vi "获取量程参数存入关键参数.vi"(7 "关键参数变更":bool, 8 "error in (no error)":errorcluster caption="错误输入（无错误）", 9 "量程":u16, 10 "flowid":u16, 11 "id":u16) -> (0 "error out":errorcluster caption="错误输出")   [LabVIEW 2016, in "斯坦道总磷.lvlib"]
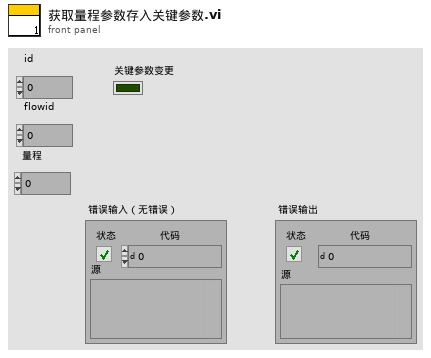
[diagram p1: front panel]
types:
  T1 = cluster{"运行模式":enum16{"维护模式", "常规模式", "应急模式", "质控模式", "性能测试"}, "质控频次":enum16{"关闭", "每天", "星期一", "星期二", "星期三", "星期四", "星期五", "星期六", "星期日"}, "空白核查时间":u16, "跨度核查时间":u16, "测量间隔":u16}
  T2 = cluster{"总磷":dbl, "总氮":dbl, "氨氮":dbl, "磷酸盐":dbl, "硝氮":dbl, "亚硝氮":dbl, "硅酸盐":dbl, "硫化物":dbl, "COD":dbl, "氟化物":dbl, "CODMn":dbl}
  T3 = cluster{"标液浓度1":dbl, "测量吸光度1":dbl, "样品1启用":bool, "标液浓度2":dbl, "测量吸光度2":dbl, "样品2启用":bool, "标液浓度3":dbl, "测量吸光度3":dbl, "样品3启用":bool, "标液浓度4":dbl, "测量吸光度4":dbl, "样品4启用":bool, "标液浓度5":dbl, "测量吸光度5":dbl, "样品5启用":bool, "模型":enum32{"线性", "多项式"}, "精度":dbl, "XY图":cluster{"X Values":dbl[], "Y Values":dbl[]}[], "拟合公式":string, "r^2":dbl, "标样一校准时间":timestamp, "标样二校准时间":timestamp, "标样三校准时间":timestamp, "标样四校准时间":timestamp, "标样五校准时间":timestamp, "二次方程":cluster{"c":dbl, "x":dbl, "x^2":dbl}, "标定时间":timestamp}
  T4 = cluster{"测量精度":u16, "检出限":dbl, "上限":dbl, "下限":dbl, "阈值（低->高）":dbl, "阈值（高->低）":dbl, "稀释度":dbl}
  T5 = typedef "SingleStepTestV3.lvlib/SingleStepTestV3.lvclass/仪器版本.ctl" = enum16{"A版", "B版", "A1版"}
  T6 = typedef "斯坦道总磷.lvlib/V3 A版外设参数.ctl" = cluster{"泵类型":u8, "进样速度":u32, "出样速度":u32, "泵阀量":u8, "阀方向":u8, "光谱仪类型":u8, "光谱采样次数":u8, "氙灯次数":u8, "B":u16, "C":u16, "D":u16, "E":u16, "B_COD":u16, "C_COD":u16, "D_COD":u16, "E_COD":u16, "G":u16, "M":u16, "N":u16, "氨氮注射泵控温下限":sgl, "氨氮注射泵控温上限":sgl, "总氮注射泵控温下限":sgl, "总氮注射泵控温上限":sgl, "消解温度下限":sgl, "消解温度上限":sgl, "加热10s限值":sgl, "KP":sgl, "KI":sgl, "KD":sgl, "高温高压阀开阀温度":sgl, "总氮x公式0":u8, "总氮x公式1":sgl, "总氮x公式2":sgl, "总磷浊度稀释系数":sgl, "总磷浊度补偿权重1":sgl, "总磷浊度补偿权重2":sgl, "盐度系数":sgl, "氨氮补偿系数1":sgl, "氨氮补偿系数2":sgl}
  T7 = typedef "斯坦道总磷.lvlib/V3 B版外设参数.ctl" = cluster{"泵类型":u8, "注射泵正常速度":u32, "注射泵慢速":u32, "阀型号":u8, "res":u8, "光谱仪类型":u8, "光谱采样次数":u8, "氙灯次数":u8, "B":u16, "C":u16, "D":u16, "E":u16, "B_COD":u16, "C_COD":u16, "D_COD":u16, "E_COD":u16, "G":u16, "M":u16, "N":u16, "降温下限":sgl, "降温上限":sgl, "恒温温度下限":sgl, "恒温温度上限":sgl, "消解温度下限":sgl, "消解温度上限":sgl, "加热10s限值":sgl, "KP":sgl, "KI":sgl, "KD":sgl, "高温高压阀开阀温度":sgl, "总氮x公式0":u8, "总氮x公式1":sgl, "总氮x公式2":sgl, "总磷浊度稀释系数":sgl, "总磷浊度补偿权重1":sgl, "总磷浊度补偿权重2":sgl, "盐度系数":sgl, "氨氮补偿系数1":sgl, "氨氮补偿系数2":sgl, "缺试剂传感器阈值":u16}
  T8 = typedef "斯坦道总磷.lvlib/V3 A1版外设参数.ctl" = cluster{"泵类型":u8, "进样速度":u32, "出样速度":u32, "泵阀量":u8, "光谱仪类型":u8, "光谱采样次数":u8, "氙灯次数":u8, "B":u16, "C":u16, "D":u16, "E":u16, "B_COD":u16, "C_COD":u16, "D_COD":u16, "E_COD":u16, "G":u16, "M":u16, "N":u16, "氨氮注射泵控温下限":sgl, "氨氮注射泵控温上限":sgl, "总氮注射泵控温下限":sgl, "总氮注射泵控温上限":sgl, "消解温度下限":sgl, "消解温度上限":sgl, "加热10s限值":sgl, "高温高压阀开阀温度":sgl, "总氮x公式0":u8, "总氮x公式1":sgl, "总氮x公式2":sgl, "总磷浊度稀释系数":sgl, "总磷浊度补偿权重1":sgl, "总磷浊度补偿权重2":sgl, "盐度系数":sgl, "氨氮补偿系数1":sgl, "氨氮补偿系数2":sgl}
  T9 = cluster{"标液浓度1":dbl, "测量吸光度1":dbl, "样品1启用":bool, "标液浓度2":dbl, "测量吸光度2":dbl, "样品2启用":bool, "标液浓度3":dbl, "测量吸光度3":dbl, "样品3启用":bool, "标液浓度4":dbl, "测量吸光度4":dbl, "样品4启用":bool, "标液浓度5":dbl, "测量吸光度5":dbl, "样品5启用":bool, "模型":enum32{"线性", "多项式"}, "精度":dbl, "XY图":cluster{"X Values":dbl[], "Y Values":dbl[]}[], "拟合公式":string, "r^2":dbl, "标样一校准时间":timestamp, "标样二校准时间":timestamp, "标样三校准时间":timestamp, "标样四校准时间":timestamp, "标样五校准时间":timestamp, "二次方程":cluster{"c":dbl, "x":dbl, "x^2":dbl}, "标定时间":timestamp}[]
  T10 = typedef "斯坦道总磷.lvlib/关键参数.ctl" = cluster{"测量量程":sgl, "测量检出限":sgl, "测量精度":sgl, "测量间隔":sgl, "消解温度":sgl, "消解时长":sgl, "三项式系数":sgl, "二次多项式系数":sgl, "曲线斜率":sgl, "曲线截距":sgl, "线性相关系数":sgl, "空白校准时间":timestamp, "标样校准时间":timestamp, "测量信号值":sgl, "稀释倍数":sgl, "空白标定系数":sgl, "量程系数":sgl}
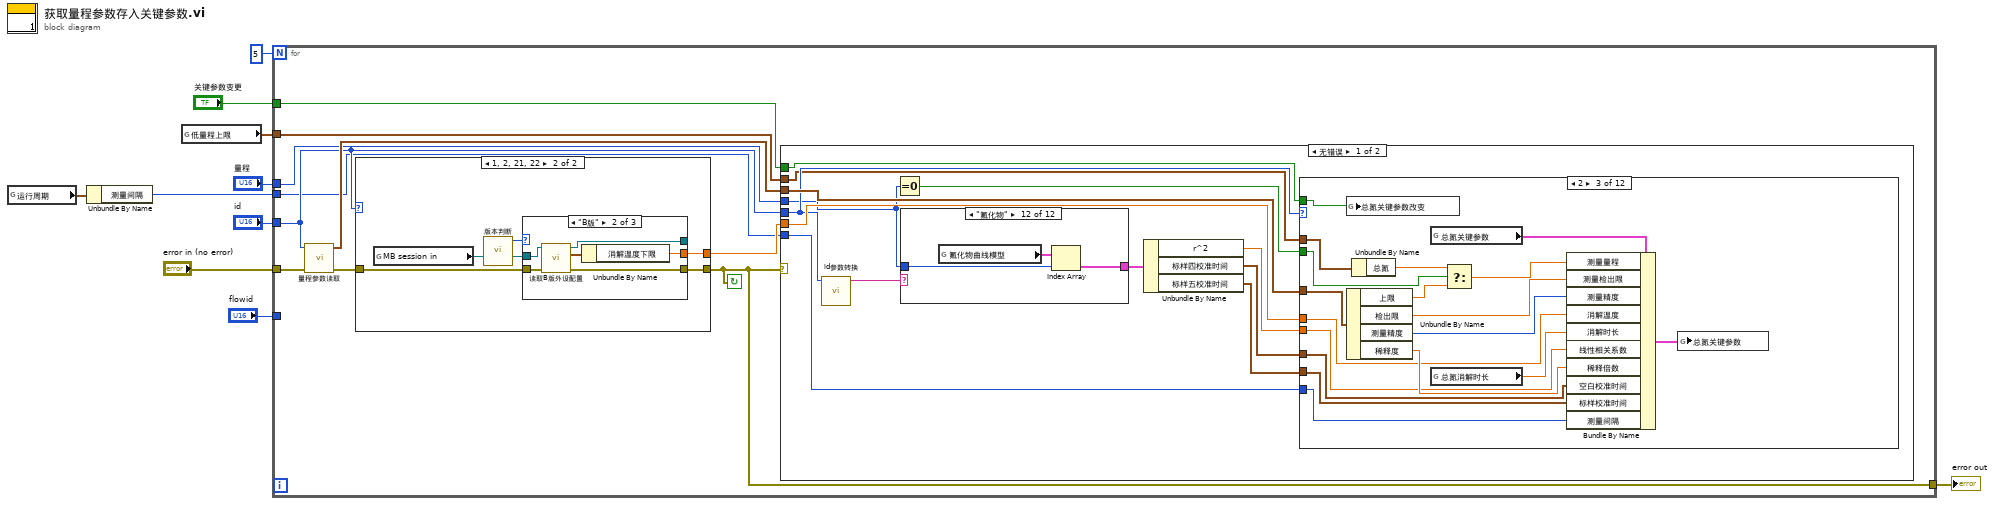
[diagram p0: block diagram]
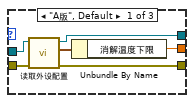
[diagram p3: hidden frame]
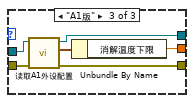
[diagram p4: hidden frame]
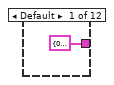
[diagram p5: hidden frame]
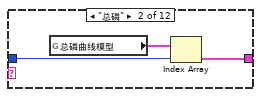
[diagram p6: hidden frame]
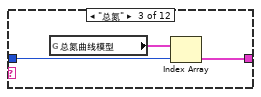
[diagram p7: hidden frame]
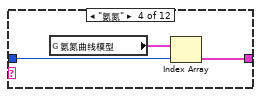
[diagram p8: hidden frame]
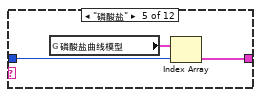
[diagram p9: hidden frame]
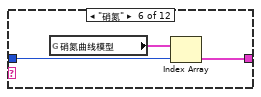
[diagram p10: hidden frame]
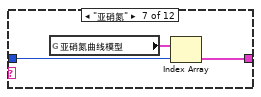
[diagram p11: hidden frame]
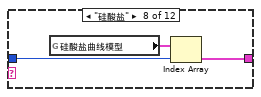
[diagram p12: hidden frame]
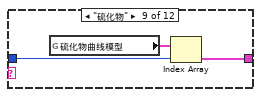
[diagram p13: hidden frame]
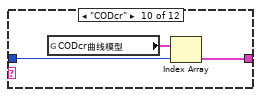
[diagram p14: hidden frame]
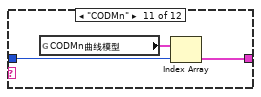
[diagram p15: hidden frame]
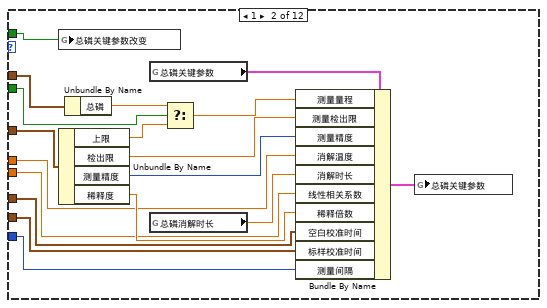
[diagram p17: hidden frame]
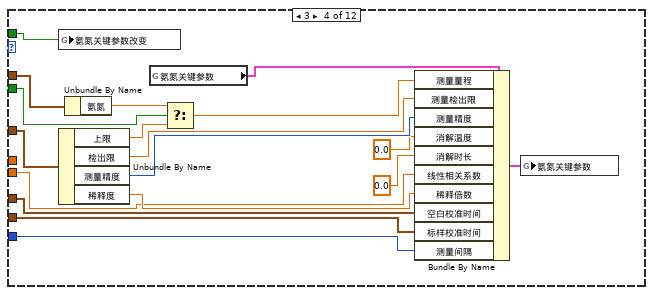
[diagram p18: hidden frame]
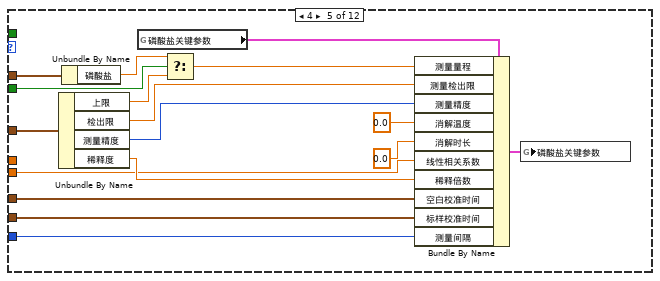
[diagram p19: hidden frame]
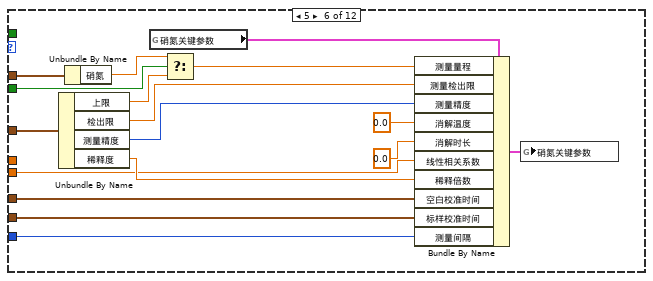
[diagram p20: hidden frame]
diagram:
  n1 = global read "总磷总氮断电保存全局变量.vi" "运行周期"() -> (w4:T1)
  n2 = Unbundle By Name(w4) -> ("测量间隔"=w3:u16)
  n3 = global read "总磷总氮断电保存全局变量.vi" "低量程上限"() -> (w2:T2)
  n4 = for {
    N: 5 -> [_]
    tunnel: "量程" -> [w18]
    tunnel: "flowid" -> [_]
    tunnel: "id" -> [w14]
    tunnel: "error in (no error)" -> [w15]
    tunnel: [w16] -> w5
    tunnel: w3 -> [w13]
    tunnel: w2 -> [w12]
    tunnel: "关键参数变更" -> [w11]
    stop <- w16 continue-if-true
    n5 = call "量程参数读取.vi"("error in (no error)"=w15, "测量参数"=w14) -> ("error out"=w17:errorcluster, "量程参数读取"=w20:T4)  [unwired: 8 in]
    n6 = case shown="1, 2, 21, 22" w14 {
      tunnel: [_ w24] -> w19
      tunnel: w17 -> [w21 w25]
      tunnel: [w21 w23] -> w16
      frame 0, Default {
      }
      frame 1, 2, 21, 22 {
        n7 = global read "VAR总磷总氮全局变量.vi" "MB session in"() -> (w26:refnum<class "MB_Master.lvclass">)
        n8 = call "版本判断.vi"() -> ("仪器版本"=w22:T5)  [unwired: 11 in]
        n9 = case shown="\"B版\"" w22 {
          tunnel: [w32 w38 w44] -> w23
          tunnel: [w30 w36 w42] -> w24
          tunnel: [w29 w35 w41] -> _
          tunnel: w26 -> [w28 w34 w40]
          tunnel: w25 -> [w27 w33 w39]
          frame "A版", Default {
            n10 = call "读取外设配置.vi"("error in (no error)"=w27, "MB session in"=w28) -> ("error out"=w32:errorcluster, "外设配置"=w31:T6, "MB session out"=w29:refnum<class "MB_Master.lvclass">)  [unwired: 7 in]
            n11 = Unbundle By Name(w31) -> ("消解温度下限"=w30:sgl)
          }
          frame "B版" {
            n12 = call "读取B版外设配置.vi"("error in (no error)"=w33, "MB session in"=w34) -> ("error out"=w38:errorcluster, "外设配置"=w37:T7, "MB session out"=w35:refnum<class "MB_Master.lvclass">)  [unwired: 7 in]
            n13 = Unbundle By Name(w37) -> ("消解温度下限"=w36:sgl)
          }
          frame "A1版" {
            n14 = call "读取A1外设配置.vi"("error in (no error)"=w39, "MB session in"=w40) -> ("error out"=w44:errorcluster, "外设配置"=w43:T8, "MB session out"=w41:refnum<class "MB_Master.lvclass">)  [unwired: 7 in]
            n15 = Unbundle By Name(w43) -> ("消解温度下限"=w42:sgl)
          }
        }
      }
    }
    n16 = case shown="无错误" w16 {
      tunnel: w20 -> [w57 _]
      tunnel: w19 -> [w56 _]
      tunnel: w14 -> [w50 _]
      tunnel: w18 -> [w47 _]
      tunnel: w13 -> [w49 _]
      tunnel: w12 -> [w48 _]
      tunnel: w11 -> [w45 _]
      frame No Error {
        n17 = call "id参数转换.vi"("id"=w50) -> ("table输出"=w55:string)  [unwired: 9 in, 1 out]
        n18 = Equal To 0?(x=w47) -> (x = 0?=w46:bool)
        n19 = case shown="\"氟化物\"" w55 {
          tunnel: w47 -> [_ w59 w62 w65 w68 w71 w74 w77 w80 w83 w86 w89]
          tunnel: [T3 {"标液浓度1"=0.0, "测量吸光度1"=0.0, "样品1启用"=FALSE, "标液浓度2"=0.0, "测量吸光度2"=0.0, "样品2启用"=FALSE, "标液浓度3"=0.0, "测量吸光度3"=0.0, "样品3启用"=FALSE, "标液浓度4"=0.0, "测量吸光度4"=0.0, "样品4启用"=FALSE, "标液浓度5"=0.0, "测量吸光度5"=0.0, "样品5启用"=FALSE, "模型"=enum."线性", "精度"=0.0, "XY图"=[], "拟合公式"="", "r^2"=0.0, "标样一校准时间"=timestamp(0 s since 1904-01-01), "标样二校准时间"=timestamp(0 s since 1904-01-01), "标样三校准时间"=timestamp(0 s since 1904-01-01), "标样四校准时间"=timestamp(0 s since 1904-01-01), "标样五校准时间"=timestamp(0 s since 1904-01-01), "二次方程"={"c"=0.0, "x"=0.0, "x^2"=0.0}, "标定时间"=timestamp(0 s since 1904-01-01)} ("总磷曲线模型") w60 w63 w66 w69 w72 w75 w78 w81 w84 w87 w90] -> w54
          frame Default {
          }
          frame "总磷" {
            n20 = global read "校准数据全局变量.vi" "总磷曲线模型"() -> (w61:T9)
            n21 = Index Array(array=w61, index=w59) -> (element=w60:T3)
          }
          frame "总氮" {
            n22 = global read "校准数据全局变量.vi" "总氮曲线模型"() -> (w64:T9)
            n23 = Index Array(array=w64, index=w62) -> (element=w63:T3)
          }
          frame "氨氮" {
            n24 = global read "校准数据全局变量.vi" "氨氮曲线模型"() -> (w67:T9)
            n25 = Index Array(array=w67, index=w65) -> (element=w66:T3)
          }
          frame "磷酸盐" {
            n26 = global read "校准数据全局变量.vi" "磷酸盐曲线模型"() -> (w70:T9)
            n27 = Index Array(array=w70, index=w68) -> (element=w69:T3)
          }
          frame "硝氮" {
            n28 = global read "校准数据全局变量.vi" "硝氮曲线模型"() -> (w73:T9)
            n29 = Index Array(array=w73, index=w71) -> (element=w72:T3)
          }
          frame "亚硝氮" {
            n30 = global read "校准数据全局变量.vi" "亚硝氮曲线模型"() -> (w76:T9)
            n31 = Index Array(array=w76, index=w74) -> (element=w75:T3)
          }
          frame "硅酸盐" {
            n32 = global read "校准数据全局变量.vi" "硅酸盐曲线模型"() -> (w79:T9)
            n33 = Index Array(array=w79, index=w77) -> (element=w78:T3)
          }
          frame "硫化物" {
            n34 = global read "校准数据全局变量.vi" "硫化物曲线模型"() -> (w82:T9)
            n35 = Index Array(array=w82, index=w80) -> (element=w81:T3)
          }
          frame "CODcr" {
            n36 = global read "校准数据全局变量.vi" "CODcr曲线模型"() -> (w85:T9)
            n37 = Index Array(array=w85, index=w83) -> (element=w84:T3)
          }
          frame "CODMn" {
            n38 = global read "校准数据全局变量.vi" "CODMn曲线模型"() -> (w88:T9)
            n39 = Index Array(array=w88, index=w86) -> (element=w87:T3)
          }
          frame "氟化物" {
            n40 = global read "校准数据全局变量.vi" "氟化物曲线模型"() -> (w91:T9)
            n41 = Index Array(array=w91, index=w89) -> (element=w90:T3)
          }
        }
        n42 = Unbundle By Name(w54) -> ("r^2"=w53:dbl, "标样四校准时间"=w52:timestamp, "标样五校准时间"=w51:timestamp)
        n43 = case shown="2" w50 {
          tunnel: w57 -> [_ w107 w125 w143 w160 w177 w194 w211 w228 w246 w264 w281]
          tunnel: w56 -> [_ w92 w110 _ _ _ _ _ _ w231 w249 w267]
          tunnel: w53 -> [_ w100 w120 w137 w152 w171 w188 w205 w220 w241 w259 w276]
          tunnel: w52 -> [_ w101 w119 w136 w154 w170 w187 w204 w222 w240 w258 w275]
          tunnel: w51 -> [_ w102 w118 w135 w153 w169 w186 w203 w221 w239 w257 w274]
          tunnel: w49 -> [_ w99 w117 w134 w151 w168 w185 w202 w219 w238 w256 w273]
          tunnel: w48 -> [_ w98 w115 w132 w149 w166 w183 w199 w217 w236 w254 w271]
          tunnel: w46 -> [_ w96 w114 w131 w148 w165 w182 w200 w216 w235 w253 w270]
          tunnel: w45 -> [_ w93 w111 w128 _ _ _ _ _ w232 w250 _]
          frame 0, Default {
          }
          frame 1 {
            n44 = global write "VAR总磷总氮全局变量.vi" "总磷关键参数改变"(w93) -> ()
            n45 = Unbundle By Name(w107) -> ("上限"=w95:dbl, "检出限"=w106:dbl, "测量精度"=w105:u16, "稀释度"=w103:dbl)
            n46 = Unbundle By Name(w98) -> ("总磷"=w97:dbl)
            n47 = global read "VAR总磷总氮全局变量.vi" "总磷关键参数"() -> (w108:T10)
            n48 = global read "总磷总氮断电保存全局变量.vi" "总磷消解时长"() -> (w104:dbl)
            n49 = Select(t=w97, s=w96, f=w95) -> (s? t:f=w94:dbl)
            n50 = Bundle By Name(cluster=w108, "测量量程"=w94, "测量检出限"=w106, "测量精度"=w105, "消解温度"=w92, "消解时长"=w104, "线性相关系数"=w100, "稀释倍数"=w103, "空白校准时间"=w101, "标样校准时间"=w102, "测量间隔"=w99) -> (w109:T10)
            n51 = global write "VAR总磷总氮全局变量.vi" "总磷关键参数"(w109) -> ()
          }
          frame 2 {
            n52 = global write "VAR总磷总氮全局变量.vi" "总氮关键参数改变"(w111) -> ()
            n53 = Unbundle By Name(w125) -> ("上限"=w113:dbl, "检出限"=w124:dbl, "测量精度"=w123:u16, "稀释度"=w121:dbl)
            n54 = Unbundle By Name(w115) -> ("总氮"=w116:dbl)
            n55 = global read "VAR总磷总氮全局变量.vi" "总氮关键参数"() -> (w126:T10)
            n56 = global read "总磷总氮断电保存全局变量.vi" "总氮消解时长"() -> (w122:dbl)
            n57 = Select(t=w116, s=w114, f=w113) -> (s? t:f=w112:dbl)
            n58 = Bundle By Name(cluster=w126, "测量量程"=w112, "测量检出限"=w124, "测量精度"=w123, "消解温度"=w110, "消解时长"=w122, "线性相关系数"=w120, "稀释倍数"=w121, "空白校准时间"=w119, "标样校准时间"=w118, "测量间隔"=w117) -> (w127:T10)
            n59 = global write "VAR总磷总氮全局变量.vi" "总氮关键参数"(w127) -> ()
          }
          frame 3 {
            n60 = global write "VAR总磷总氮全局变量.vi" "氨氮关键参数改变"(w128) -> ()
            n61 = Unbundle By Name(w143) -> ("上限"=w130:dbl, "检出限"=w142:dbl, "测量精度"=w141:u16, "稀释度"=w140:dbl)
            n62 = Unbundle By Name(w132) -> ("氨氮"=w133:dbl)
            n63 = global read "VAR总磷总氮全局变量.vi" "氨氮关键参数"() -> (w144:T10)
            n64 = Select(t=w133, s=w131, f=w130) -> (s? t:f=w129:dbl)
            n65 = Bundle By Name(cluster=w144, "测量量程"=w129, "测量检出限"=w142, "测量精度"=w141, "消解温度"=sgl 0.0, "消解时长"=sgl 0.0, "线性相关系数"=w137, "稀释倍数"=w140, "空白校准时间"=w136, "标样校准时间"=w135, "测量间隔"=w134) -> (w145:T10)
            n66 = global write "VAR总磷总氮全局变量.vi" "氨氮关键参数"(w145) -> ()
          }
          frame 4 {
            n67 = Unbundle By Name(w160) -> ("上限"=w147:dbl, "检出限"=w159:dbl, "测量精度"=w158:u16, "稀释度"=w157:dbl)
            n68 = Unbundle By Name(w149) -> ("磷酸盐"=w150:dbl)
            n69 = global read "VAR总磷总氮全局变量.vi" "磷酸盐关键参数"() -> (w161:T10)
            n70 = Select(t=w150, s=w148, f=w147) -> (s? t:f=w146:dbl)
            n71 = Bundle By Name(cluster=w161, "测量量程"=w146, "测量检出限"=w159, "测量精度"=w158, "消解温度"=sgl 0.0, "消解时长"=sgl 0.0, "线性相关系数"=w152, "稀释倍数"=w157, "空白校准时间"=w154, "标样校准时间"=w153, "测量间隔"=w151) -> (w162:T10)
            n72 = global write "VAR总磷总氮全局变量.vi" "磷酸盐关键参数"(w162) -> ()
          }
          frame 5 {
            n73 = Unbundle By Name(w177) -> ("上限"=w164:dbl, "检出限"=w176:dbl, "测量精度"=w175:u16, "稀释度"=w174:dbl)
            n74 = Unbundle By Name(w166) -> ("硝氮"=w167:dbl)
            n75 = global read "VAR总磷总氮全局变量.vi" "硝氮关键参数"() -> (w178:T10)
            n76 = Select(t=w167, s=w165, f=w164) -> (s? t:f=w163:dbl)
            n77 = Bundle By Name(cluster=w178, "测量量程"=w163, "测量检出限"=w176, "测量精度"=w175, "消解温度"=sgl 0.0, "消解时长"=sgl 0.0, "线性相关系数"=w171, "稀释倍数"=w174, "空白校准时间"=w170, "标样校准时间"=w169, "测量间隔"=w168) -> (w179:T10)
            n78 = global write "VAR总磷总氮全局变量.vi" "硝氮关键参数"(w179) -> ()
          }
          frame 6 {
            n79 = Unbundle By Name(w194) -> ("上限"=w181:dbl, "检出限"=w193:dbl, "测量精度"=w192:u16, "稀释度"=w191:dbl)
            n80 = Unbundle By Name(w183) -> ("亚硝氮"=w184:dbl)
            n81 = global read "VAR总磷总氮全局变量.vi" "亚硝氮关键参数"() -> (w195:T10)
            n82 = Select(t=w184, s=w182, f=w181) -> (s? t:f=w180:dbl)
            n83 = Bundle By Name(cluster=w195, "测量量程"=w180, "测量检出限"=w193, "测量精度"=w192, "消解温度"=sgl 0.0, "消解时长"=sgl 0.0, "线性相关系数"=w188, "稀释倍数"=w191, "空白校准时间"=w187, "标样校准时间"=w186, "测量间隔"=w185) -> (w196:T10)
            n84 = global write "VAR总磷总氮全局变量.vi" "亚硝氮关键参数"(w196) -> ()
          }
          frame 7 {
            n85 = Unbundle By Name(w211) -> ("上限"=w198:dbl, "检出限"=w210:dbl, "测量精度"=w209:u16, "稀释度"=w208:dbl)
            n86 = Unbundle By Name(w199) -> ("硅酸盐"=w201:dbl)
            n87 = global read "VAR总磷总氮全局变量.vi" "硅酸盐关键参数"() -> (w212:T10)
            n88 = Select(t=w201, s=w200, f=w198) -> (s? t:f=w197:dbl)
            n89 = Bundle By Name(cluster=w212, "测量量程"=w197, "测量检出限"=w210, "测量精度"=w209, "消解温度"=sgl 0.0, "消解时长"=sgl 0.0, "线性相关系数"=w205, "稀释倍数"=w208, "空白校准时间"=w204, "标样校准时间"=w203, "测量间隔"=w202) -> (w213:T10)
            n90 = global write "VAR总磷总氮全局变量.vi" "硅酸盐关键参数"(w213) -> ()
          }
          frame 8 {
            n91 = Unbundle By Name(w228) -> ("上限"=w215:dbl, "检出限"=w227:dbl, "测量精度"=w226:u16, "稀释度"=w225:dbl)
            n92 = Unbundle By Name(w217) -> ("硫化物"=w218:dbl)
            n93 = global read "VAR总磷总氮全局变量.vi" "硫化物关键参数"() -> (w229:T10)
            n94 = Select(t=w218, s=w216, f=w215) -> (s? t:f=w214:dbl)
            n95 = Bundle By Name(cluster=w229, "测量量程"=w214, "测量检出限"=w227, "测量精度"=w226, "消解温度"=sgl 0.0, "消解时长"=sgl 0.0, "线性相关系数"=w220, "稀释倍数"=w225, "空白校准时间"=w222, "标样校准时间"=w221, "测量间隔"=w219) -> (w230:T10)
            n96 = global write "VAR总磷总氮全局变量.vi" "硫化物关键参数"(w230) -> ()
          }
          frame 22 {
            n97 = global write "VAR总磷总氮全局变量.vi" "CODCr关键参数改变"(w232) -> ()
            n98 = Unbundle By Name(w246) -> ("上限"=w234:dbl, "检出限"=w245:dbl, "测量精度"=w244:u16, "稀释度"=w243:dbl)
            n99 = Unbundle By Name(w236) -> ("亚硝氮"=w237:dbl)
            n100 = global read "VAR总磷总氮全局变量.vi" "CODcr关键参数"() -> (w247:T10)
            n101 = global read "总磷总氮断电保存全局变量.vi" "CODcr消解时长"() -> (w242:dbl)
            n102 = Select(t=w237, s=w235, f=w234) -> (s? t:f=w233:dbl)
            n103 = Bundle By Name(cluster=w247, "测量量程"=w233, "测量检出限"=w245, "测量精度"=w244, "消解温度"=w231, "消解时长"=w242, "线性相关系数"=w241, "稀释倍数"=w243, "空白校准时间"=w240, "标样校准时间"=w239, "测量间隔"=w238) -> (w248:T10)
            n104 = global write "VAR总磷总氮全局变量.vi" "CODcr关键参数"(w248) -> ()
          }
          frame 21 {
            n105 = global write "VAR总磷总氮全局变量.vi" "CODmn关键参数改变"(w250) -> ()
            n106 = Unbundle By Name(w264) -> ("上限"=w252:dbl, "检出限"=w263:dbl, "测量精度"=w262:u16, "稀释度"=w261:dbl)
            n107 = Unbundle By Name(w254) -> ("CODMn"=w255:dbl)
            n108 = global read "VAR总磷总氮全局变量.vi" "CODMn关键参数"() -> (w265:T10)
            n109 = global read "总磷总氮断电保存全局变量.vi" "CODmn消解时长"() -> (w260:dbl)
            n110 = Select(t=w255, s=w253, f=w252) -> (s? t:f=w251:dbl)
            n111 = Bundle By Name(cluster=w265, "测量量程"=w251, "测量检出限"=w263, "测量精度"=w262, "消解温度"=w249, "消解时长"=w260, "线性相关系数"=w259, "稀释倍数"=w261, "空白校准时间"=w258, "标样校准时间"=w257, "测量间隔"=w256) -> (w266:T10)
            n112 = global write "VAR总磷总氮全局变量.vi" "CODMn关键参数"(w266) -> ()
          }
          frame 50 {
            n113 = Unbundle By Name(w281) -> ("上限"=w269:dbl, "检出限"=w280:dbl, "测量精度"=w279:u16, "稀释度"=w278:dbl)
            n114 = Unbundle By Name(w271) -> ("氟化物"=w272:dbl)
            n115 = global read "总磷总氮断电保存全局变量.vi" "CODmn消解时长"() -> (w277:dbl)
            n116 = global read "VAR总磷总氮全局变量.vi" "氟化物关键参数"() -> (w282:T10)
            n117 = Select(t=w272, s=w270, f=w269) -> (s? t:f=w268:dbl)
            n118 = Bundle By Name(cluster=w282, "测量量程"=w268, "测量检出限"=w280, "测量精度"=w279, "消解温度"=w267, "消解时长"=w277, "线性相关系数"=w276, "稀释倍数"=w278, "空白校准时间"=w275, "标样校准时间"=w274, "测量间隔"=w273) -> (w283:T10)
            n119 = global write "VAR总磷总氮全局变量.vi" "氟化物关键参数"(w283) -> ()
          }
        }
      }
      frame Error {
      }
    }
  }
  "error out" <- w5
